vi "Get File Name.vi"(8 "error in":errorcluster, 11 "reference in":refnum<class "Electronic Datasheet.lvclass">) -> (0 "error out":errorcluster, 2 "File Name":string, 3 "reference out":refnum<class "Electronic Datasheet.lvclass">)   [LabVIEW 2024, in "Electronic Datasheet.lvlib" / "Electronic Datasheet.lvclass"]
uses:
  Electronic Datasheet/Electronic Datasheet.lvclass
  Electronic Datasheet/Electronic Datasheet.lvclass/Electronic Datasheet.ctl
  File Info/File Info.lvclass
  <userlib>/_OpenG.lib/lvdata/lvdata.llb/openg_variant.lvlib
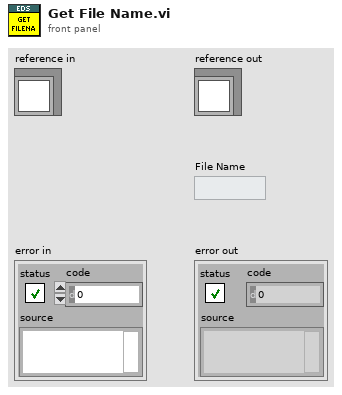
[diagram p1: front panel]
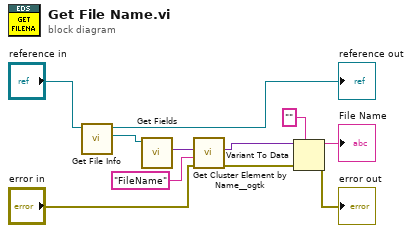
[diagram p0: block diagram]
diagram:
  n1 = call "Get File Info.vi"("reference in"="reference in") -> ("File Info"=w9:refnum<class "File Info.lvclass">, "reference out"=→"reference out":refnum<class "Electronic Datasheet.lvclass">)  [unwired: 9 in]
  n2 = call-dynamic "Get Fields.vi"("File Info in"=w9) -> ("Fields"=w8:variant)  [unwired: 9 in, 1 out]
  n3 = call <userlib>:"Get Cluster Element by Name__ogtk.vi"("error in (no error)"="error in", "Element Name"="FileName" ("element"), "Cluster"=w8) -> ("error out"=w5:errorcluster, "VElement"=w3:variant)  [unwired: 6 in, 1 out]
  n4 = Variant To Data(error in=w5, type="", Variant=w3) -> (data=→"File Name":string, error out=→"error out":errorcluster)
